vi "Time Control.vi"() -> ()   [LabVIEW 2013]
panel:
  in  "Time Target (s)":dbl=1.0
  in  "stop":bool
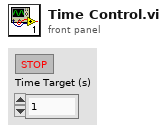
[diagram p1: front panel]
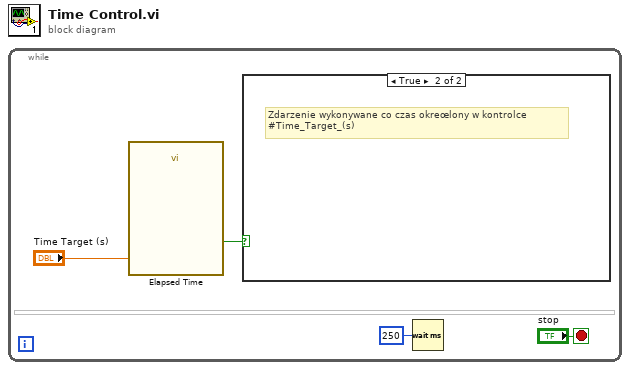
[diagram p0: block diagram]
diagram:
  n1 = while {
    stop <- "stop" stop-if-true
    n2 = call "Elapsed Time"("Time Target (s)"="Time Target (s)") -> ("Time has Elapsed"=w3:bool)  [unwired: 11 in, 7 out]
    n3 = case shown="True" w3 {
      frame False {
      }
      frame True {
        # "Zdarzenie wykonywane co czas okreœlony w kontrolce #Time_Target_(s)"
      }
    }
    n4 = Wait (ms)(milliseconds to wait=u32 250) -> ()  [unwired: 1 out]
  }
